vi "FA_ApplyINItags.vi"(8 "error in (no error)":errorcluster, 11 "INI":T1) -> (0 "error out":errorcluster)   [LabVIEW 2013]
uses:
  FA_INI.ctl
  <vilib>/Utility/config.llb/Write Key (String).vi
  <vilib>/Utility/config.llb/NI_LVConfig.lvlib
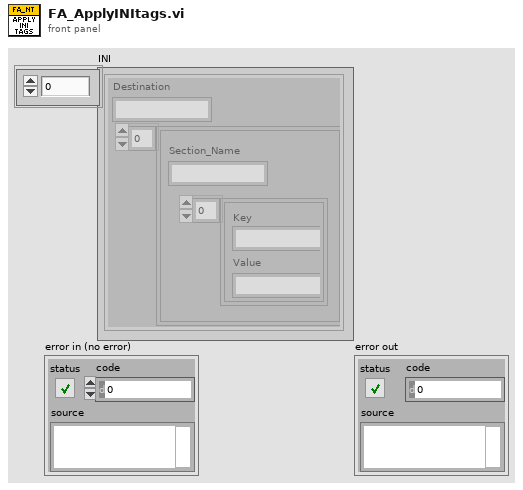
[diagram p1: front panel]
types:
  T1 = typedef "FA_INI.ctl" = cluster{"Destination":string, "Section":cluster{"Section_Name":string, "Token":cluster{"Key":string, "Value":string}[]}[]}[]
  T2 = cluster{"Section_Name":string, "Token":cluster{"Key":string, "Value":string}[]}[]
  T3 = typedef "NI_LVConfig.lvlib/Config Data RefNum.ctl" = refnum<k1>
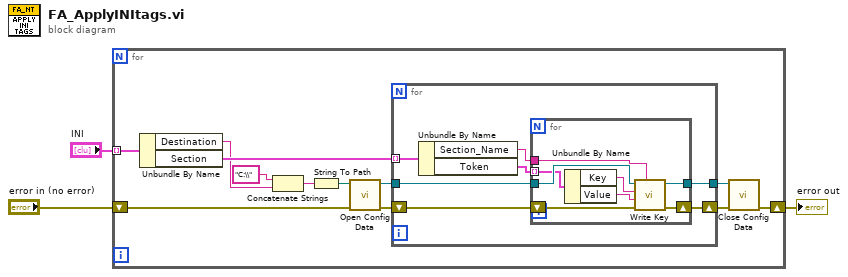
[diagram p0: block diagram]
diagram:
  n1 = for {
    tunnel: "INI" -> [w15] mode=indexing
    shift-right: [w8] -> w3
    shift-left: "error in (no error)" -> [w7]
    n2 = Unbundle By Name(w15) -> ("Destination"=w5:string, "Section"=w14:T2)
    n3 = Concatenate Strings("C:\\" ("string"), w5) -> (w6:string)
    n4 = String To Path(string=w6) -> (path=w13:path)
    n5 = call <vilib>:"Open Config Data.vi"("error in (no error)"=w7, "configuration file path"=w13) -> ("error out"=w11:errorcluster, "refnum"=w12:T3)  [unwired: 7 in, 1 out]
    n6 = for {
      tunnel: w14 -> [w20] mode=indexing
      tunnel: w12 -> [w22]
      shift-right: [w18] -> w10
      shift-left: w11 -> [w17]
      tunnel: [w21] -> w9
      n7 = Unbundle By Name(w20) -> ("Section_Name"=w19:string, "Token"=w16:cluster{"Key":string, "Value":string}[])
      n8 = for {
        tunnel: w22 -> [w30]
        tunnel: [w27] -> w21
        tunnel: w19 -> [w25]
        shift-right: [w29] -> w18
        shift-left: w17 -> [w24]
        tunnel: w16 -> [w23] mode=indexing
        n9 = Unbundle By Name(w23) -> ("Key"=w28:string, "Value"=w26:string)
        n10 = call-poly <vilib>:"Write Key.vi"("section"=w25, "error in (no error)"=w24, "value"=w26, "key"=w28, "refnum"=w30) -> ("error out"=w29:errorcluster, "refnum out"=w27:T3)  [unwired: 4 in, 1 out]
      }
    }
    n11 = call <vilib>:"Close Config Data.vi"("error in (no error)"=w10, "refnum"=w9) -> ("error out"=w8:errorcluster)  [unwired: 8 in, 1 out]
  }
  "error out" <- w3
